vi "Create Event Topics.vi"() -> (0 "error out":errorcluster, 3 "appended array":string[][](array[string]))   [LabVIEW 2013, in "FRCts20_SNS.lvlib"]
uses:
  FRCts20_SNS.lvlib
  Perforce/penguin_1666/mblack_PerforceWin/lvdotcom/source/aws-toolkit/r1/trunk/SNS/VI Source/AWS SNS Class/AWS_SNS.lvclass
  <vilib>/National Instruments/LabVIEW Interface for Amazon S3/Typedefs/AMZ_S3_AWS Credentials.ctl
  <vilib>/National Instruments/LabVIEW Interface for Amazon S3/LV Interface for Amazon S3.lvlib
  Perforce/penguin_1666/mblack_PerforceWin/lvdotcom/source/aws-toolkit/r1/trunk/SNS/VI Source/Public Typedefs/AWS_SNS SetTopicAttributes.ctl
  Perforce/penguin_1666/mblack_PerforceWin/lvdotcom/source/aws-toolkit/r1/trunk/SNS/VI Source/AWS_SNS.lvlib
  Perforce/penguin_1666/mblack_PerforceWin/lvdotcom/source/aws-toolkit/r1/trunk/SNS/VI Source/Public Typedefs/AWS_SNS CreateTopicParameters.ctl
  <vilib>/Utility/file.llb/Read From Spreadsheet File (string).vi
panel:
  out "TopicArn":string
  out "resulting string":string
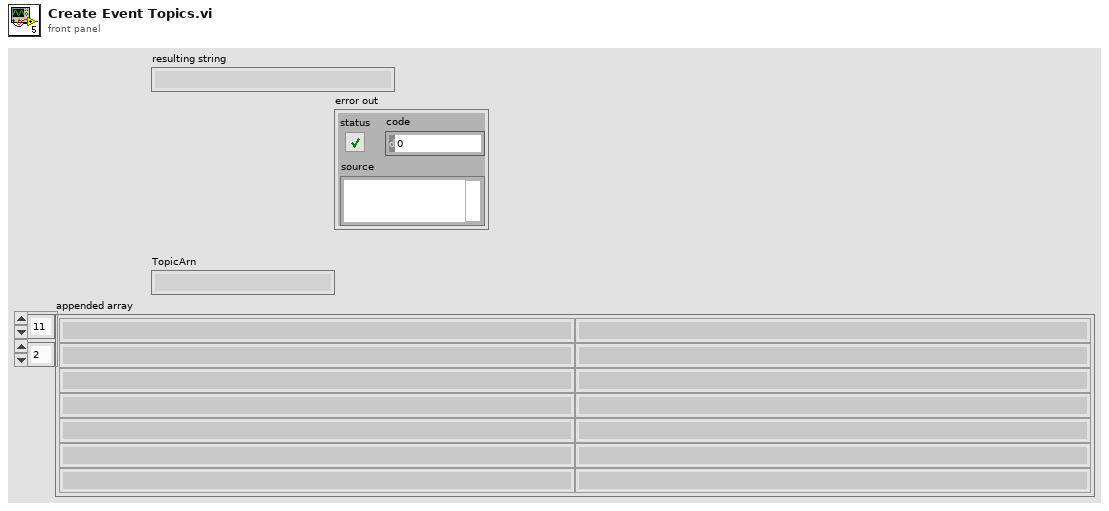
[diagram p1: front panel]
types:
  T1 = typedef "AWS_SNS.lvlib/AWS_SNS CreateTopicParameters.ctl" = string
  T2 = typedef "LV Interface for Amazon S3.lvlib/AMZ_S3_AWS Credentials.ctl" = cluster{"Access Key":string, "Secret Key":string}
  T3 = typedef "AWS_SNS.lvlib/AWS_SNS SetTopicAttributes.ctl" = cluster{"AttributeName":string, "AttributeValue":string, "TopicArn":string}
  T4 = typedef "AWS_SNS.lvlib/CreateTopicResult.ctl" = string
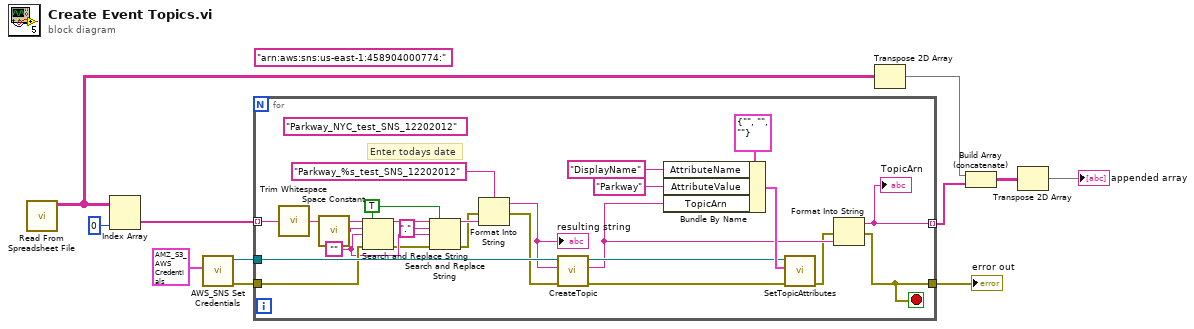
[diagram p0: block diagram]
diagram:
  (unwired) T1 "arn:aws:sns:us-east-1:458904000774:" ("CreateTopic Parameters")
  n1 = call-poly <vilib>:"Read From Spreadsheet File.vi"() -> ("all rows"=w4:string[][])  [unwired: 7 in, 4 out]
  n2 = Index Array(array=w4, index (col)=0 ("disabled index (col)")) -> (element=w6:string[])  [unwired: 1 in]
  n3 = call "AWS_SNS Set Credentials.vi"("AWS Credentials"=T2 {"Access Key"="AKIAI4UOFGXQQ2XM3KTQ", "Secret Key"="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"} ("AWS Credentials in")) -> ("error out"=w8:errorcluster, "AWS_SNS.lvlib:AWS_SNS.lvclass"=w9:refnum<class "AWS_SNS.lvclass">)  [unwired: 9 in]
  n4 = for {
    tunnel: w6 -> [w30] mode=indexing
    tunnel: w9 -> [w31]
    tunnel: w8 -> [w25]
    tunnel: [w12] -> w7
    tunnel: [w14] -> w5 mode=indexing
    stop <- w12 stop-if-true
    w22 = ""
    w20 = TRUE ("replace all? (F)")
    (unwired) T1 "Parkway_NYC_test_SNS_12202012" ("CreateTopic Parameters")
    # "Enter todays date"
    n5 = call <vilib>:"Trim Whitespace.vi"("string"=w30) -> ("trimmed string"=w27:string)  [unwired: 1 in]
    n6 = call <vilib>:"Space Constant.vi"() -> ("String"=w26:string)
    n7 = Search and Replace String(replace all?=w20, input string=w27, search string=w26, replace string=w22, error in=w25) -> (result string=w23:string, error out=w17:errorcluster)  [unwired: 3 in, 2 out]
    n8 = Search and Replace String(replace all?=w20, input string=w23, search string=".", replace string=w22, error in=w17) -> (result string=w19:string, error out=w16:errorcluster)  [unwired: 3 in, 2 out]
    n9 = Format Into String(format string="Parkway_%s_test_SNS_12202012", error in=w16, w19) -> (resulting string=w28:string, error out=w24:errorcluster)  [unwired: 1 in]
    "resulting string" <- w28
    n10 = call-dynamic "CreateTopic.vi"("error in (no error)"=w24, "CreateTopic Parameters"=w28, "AWS_SNS in"=w31) -> ("error out"=w33:errorcluster, "TopicArn"=w15:T4, "AWS_SNS out"=w32:refnum<class "AWS_SNS.lvclass">)  [unwired: 6 in]
    n11 = Bundle By Name(cluster=T3 {"AttributeName"="", "AttributeValue"="", "TopicArn"=""} ("SetTopicAttributes Parameters"), "AttributeName"="DisplayName", "AttributeValue"="Parkway" ("trimmed string"), "TopicArn"=w15) -> (w35:T3)
    n12 = call-dynamic "SetTopicAttributes.vi"("error in (no error)"=w33, "SetTopicAttributes Parameters"=w35, "AWS_SNS.lvlib:AWS_SNS.lvclass"=w32) -> ("error out"=w13:errorcluster)  [unwired: 7 in, 1 out]
    n13 = Format Into String(error in=w13, w15) -> (resulting string=w14:string, error out=w12:errorcluster)  [unwired: 2 in]
    "TopicArn" <- w14
  }
  "error out" <- w7
  n14 = Transpose 2D Array(2D array=w4) -> (transposed array=w3:string[][])
  n15 = Build Array (concatenate)(w3, w5) -> (w2:string[][])
  n16 = Transpose 2D Array(2D array=w2) -> (transposed array=→"appended array":string[][])
